vi "Get Qualified Name.vi"(8 "error in (no error)":errorcluster, 10 "separator (dot)":string caption="separator", 11 "SMO":refnum<class "SMO.lvclass">) -> (0 "error out":errorcluster, 2 "Qualified Name":string, 3 "SMO out":refnum<class "SMO.lvclass">)   [LabVIEW 2019, in "SMO.lvclass"]
doc: "JKI State Machine Objects (SMO) 1.3.0.56\nJKI - JKI\nCopyright (c) 2017, JKI"
uses:
  SMO.lvclass
  Support/Attribute.Owner/Attribute.Owner.lvclass
  C:/Users/Patrick/Documents/GitHub/Test (LV2019)/lv-venv/lv.lib/vi.lib/JKI/JKI SMO/Support/Attribute/Attribute.lvclass
  Support/Attribute.Owner/Attribute.Owner.lvclass/Attribute.Owner.ctl
  Support/Attribute/Attribute.lvclass
panel:
  # "This method is deprecated but kept for\nbackward-compatibility.\nUse the \"GetQualifiedName.vi\" method instead of \"Get Qualified Name.vi\""
  # "For instructions on how to use the JKI State Machine Objects, examples and video tutorials, visit:\nhttp://jki.net/state-machine-objects/\n\nJKI State Machine Objects™\nhttp://jki.net/state-machine-objects/\nCopyright (C) 2005-2015, JKI <info@jki.net>\nALL RIGHTS RESERVED"
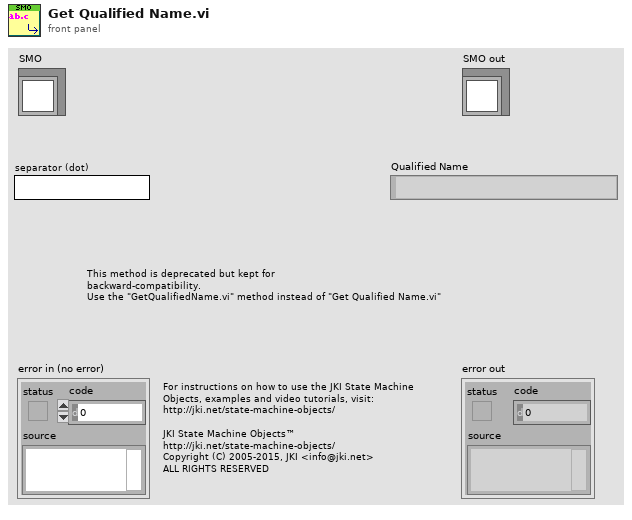
[diagram p1: front panel]
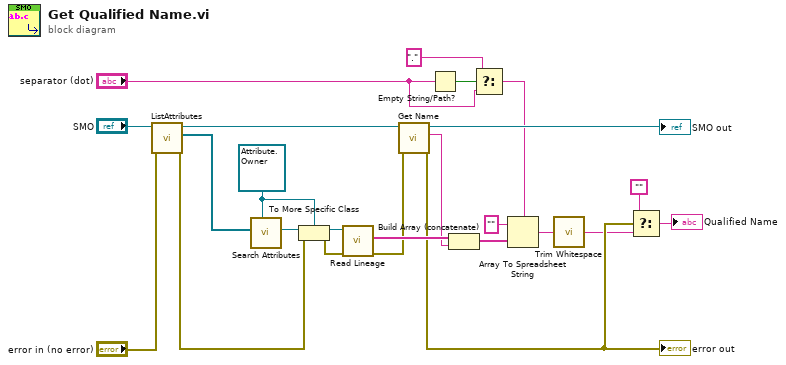
[diagram p0: block diagram]
diagram:
  w18 = refnum<class "Attribute.Owner.lvclass"> refnum ("Attribute.Owner.lvclass")
  n1 = call "ListAttributes.vi"("error in (no error)"="error in (no error)", "SMO in"="SMO") -> ("error out"=w10:errorcluster, "[Attributes]"=w20:refnum<class "Attribute.lvclass">[], "SMO out"=w15:refnum<class "SMO.lvclass">)  [unwired: 7 in]
  n2 = call "Search Attributes.vi"("Attribute type"=w18, "[Attributes]"=w20) -> ("Attribute out"=w24:refnum<class "Attribute.lvclass">)  [unwired: 8 in, 1 out]
  n3 = To More Specific Class(target class=w18, reference=w24, error in=w10) -> (specific class reference=w17:refnum<class "Attribute.Owner.lvclass">, error out=w16:errorcluster)
  n4 = call "Read Lineage.vi"("error in (no error)"=w16, "Attribute.Owner in"=w17) -> ("error out"=w11:errorcluster, "Lineage"=w13:string[])  [unwired: 7 in, 1 out]
  n5 = call "Get Name.vi"("error in (no error)"=w11, "SMO"=w15) -> ("error out"=w9:errorcluster, "Name"=w12:string, "SMO out"=→"SMO out":refnum<class "SMO.lvclass">)  [unwired: 7 in]
  "error out" <- w9
  n6 = Empty String/Path?(string/path="separator (dot)") -> (empty?=w4:bool)
  n7 = Build Array (concatenate)(w13, w12) -> (w8:string[])
  n8 = Select(t="." ("delimiter (Tab)"), s=w4, f="separator (dot)") -> (s? t:f=w1:string)
  n9 = Array To Spreadsheet String(delimiter (Tab)=w1, array=w8, 3:"" ("format string")) -> (spreadsheet string=w6:string)
  n10 = call <vilib>:"Trim Whitespace.vi"("string"=w6) -> ("trimmed string"=w5:string)  [unwired: 1 in]
  n11 = Select(t="", s=w9, f=w5) -> (s? t:f=→"Qualified Name":string)
